vi "Persist Variables.vi"(11 "Path":path) -> ()   [LabVIEW 2017]
uses:
  <vilib>/Rock Robotics/Network Tables/Make Table Operation.ctl
  <vilib>/Utility/config.llb/Write Key (String).vi
  <vilib>/Utility/config.llb/NI_LVConfig.lvlib
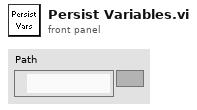
[diagram p1: front panel]
types:
  T1 = enum16{"Add", "Remove", "Clear", "Init", "Retrieve"}
  T2 = typedef "Field ID.ctl" = i32
  T3 = enum16{"Update Field", "Read Field", "Assign Field", "Remove All", "Set Persistence", "Clear Persistence"}
  T4 = typedef "Make Table Operation.ctl" = enum16{"Get or Add Field", "Get Field or Add Temp", "Replace Temp ID", "Get Field ID - No Add", "Get Table Field IDs", "Get Field ID Info", "Move Field to Temp", "Validate", "Remove Field", "Remove All"}
  T5 = typedef "NI_LVConfig.lvlib/Config Data RefNum.ctl" = refnum<k1>
  T6 = typedef "Field Data.ctl" = cluster{"Dbl":dbl, "String":string, "Type":T7, "Boolean":bool, "Sequence #":T8, "Flags":u8}
  T7 = typedef "Field Type.ctl" = enum8{"Invalid", "Bool", "Numeric", "String", "Raw", "Boolean Array", "Numeric Array", "String Array", "RPC"}
  T8 = typedef "Sequence.ctl" = u16
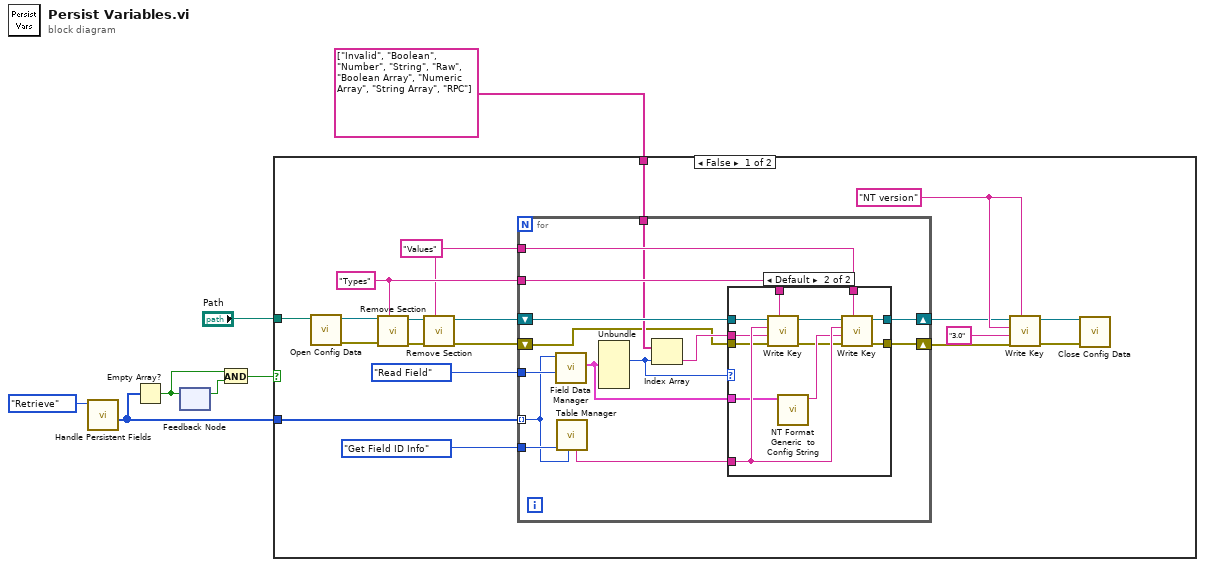
[diagram p0: block diagram]
diagram:
  n1 = call <vilib>:"Handle Persistent Fields.vi"("Operation"=T1."Retrieve") -> ("Field IDs out"=w4:T2[])  [unwired: 10 in]
  n2 = Empty Array?(array=w4) -> (empty?=w3:bool)
  n3 = feedback-in #1(w3) -> ()
  n4 = feedback #1() -> (w2:bool)  [unwired: 1 in]
  n5 = And(x=w3, y=w2) -> (x .and. y?=w1:bool)
  n6 = case shown="False" w1 {
    tunnel: w4 -> [w26 _]
    tunnel: string[] ["Invalid", "Boolean", "Number", "String", "Raw", "Boolean Array", "Numeric Array", "String Array", "RPC"] -> [w20 _]
    tunnel: "Path" -> [w16 _]
    frame False {
      w19 = "NT version" ("section")
      w21 = "Values" ("section")
      w22 = "Types" ("section")
      n7 = call <vilib>:"Open Config Data.vi"("configuration file path"=w16) -> ("error out"=w13:errorcluster, "refnum"=w15:T5)  [unwired: 8 in, 1 out]
      n8 = call <vilib>:"Remove Section.vi"("section"=w22, "error in (no error)"=w13, "refnum"=w15) -> ("error out"=w12:errorcluster, "refnum out"=w24:T5)  [unwired: 6 in, 1 out]
      n9 = call <vilib>:"Remove Section.vi"("section"=w21, "error in (no error)"=w12, "refnum"=w24) -> ("error out"=w11:errorcluster, "refnum out"=w23:T5)  [unwired: 6 in, 1 out]
      n10 = for {
        tunnel: w26 -> [w38] mode=indexing
        tunnel: T3."Read Field" ("Operation") -> [w40]
        tunnel: Make_Table_Operation."Get Field ID Info" ("Operation") -> [w39]
        shift-right: [w36] -> w18
        shift-left: w23 -> [w37]
        tunnel: w22 -> [w35]
        tunnel: w21 -> [w34]
        tunnel: w20 -> [w32]
        shift-right: [w28] -> w10
        shift-left: w11 -> [w27]
        n11 = call <vilib>:"Field Data Manager.vi"("Operation"=w40, "Field ID"=w38) -> ("Field Value Out"=w30:T6)  [unwired: 8 in, 1 out]
        n12 = call <vilib>:"Table Manager.vi"("Entry ID in"=w38, "Operation"=w39) -> ("Entry Name"=w33:string)  [unwired: 6 in, 3 out]
        n13 = Unbundle(w30) -> ("Type"=w29:T7)  [unwired: 5 out]
        n14 = Index Array(array=w32, index=w29) -> (element=w31:string)
        n15 = case shown="Default" w29 {
          tunnel: w37 -> [w42 w54]
          tunnel: [w42 w52] -> w36
          tunnel: w35 -> [_ w51]
          tunnel: w34 -> [_ w50]
          tunnel: w33 -> [_ w49]
          tunnel: w31 -> [_ w48]
          tunnel: w30 -> [_ w47]
          tunnel: [w41 w45] -> w28
          tunnel: w27 -> [w41 w43]
          frame "Invalid", "RPC" {
          }
          frame Default {
            n16 = call-poly <vilib>:"Write Key.vi"("section"=w51, "error in (no error)"=w43, "value"=w48, "key"=w49, "refnum"=w54) -> ("error out"=w44:errorcluster, "refnum out"=w53:T5)  [unwired: 4 in, 1 out]
            n17 = call <vilib>:"NT Format Generic  to Config String.vi"("Field Value"=w47) -> ("String"=w46:string)  [unwired: 10 in]
            n18 = call-poly <vilib>:"Write Key.vi"("section"=w50, "error in (no error)"=w44, "value"=w46, "key"=w49, "refnum"=w53) -> ("error out"=w45:errorcluster, "refnum out"=w52:T5)  [unwired: 4 in, 1 out]
          }
        }
      }
      n19 = call-poly <vilib>:"Write Key.vi"("section"=w19, "error in (no error)"=w10, "value"="3.0" ("section"), "key"=w19, "refnum"=w18) -> ("error out"=w9:errorcluster, "refnum out"=w14:T5)  [unwired: 4 in, 1 out]
      n20 = call <vilib>:"Close Config Data.vi"("error in (no error)"=w9, "refnum"=w14) -> ()  [unwired: 8 in, 2 out]
    }
    frame True {
    }
  }
